vi "RSZVB Select Y-Parameters.vi"(4 "Out Mode (0: Single-ended (for unbalanced ports))":u16(ring) items=["Single-ended", "Differential", "Common"], 5 "In Port (1)":i32=1, 6 "In Mode (0: Single-ended (for unbalanced ports))":u16(ring) items=["Single-ended", "Differential", "Common"], 7 "Out Port (1)":i32=1, 8 "error in (no error)":errorcluster {"code" format="%.0x"}, 9 "Trace Name (Trc1)":string="Trc1", 10 "Channel (1)":i32=1, 11 "VISA session":refnum<visa-resource-name>) -> (0 "error out":errorcluster {"code" format="%.0x"}, 3 "dup VISA session":refnum<visa-resource-name>)   [LabVIEW 2011]
doc: "This VI select short-circuit Y-parameters for multiport measurements (including the 2-port Y-parameters) or mixed mode Y-parameters. All possible combinations of mixed mode parameters (e.g. Yss, Ycs, Yds, Ydd,...) are provided.\n\nAssigns a measurement parameter to an existing trace or creates a trace and assigns a channel number, a name and a measurement parameter to it. The trace is not displayed.\n\nMixed mode parameters are used to distinguish the following three port modes: \n\nSingle-ended (for unbalanced ports)\nDifferential mode (for balanced ports)\nCommon mode (for balanced ports) \n\nThe notation of a general Y-parameter is Y<mout><min><out><in>, where <mout> and <min> denote the output and input port modes, <out> and <in> denote the output and input port numbers.\n\nThe selected modes must be compatible with the port configuration. If an attempt is made to select an incompatible parameter (e.g. a single-ended parameter for a balanced port), the analyzer displays an error message.\n\nRemote-control command(s):\nCALCulate<Ch>:PARameter:SDEFine '<string>', 'Y11' | 'Y12' | 'Y21' | 'Y22' | ...\nCALCulate<Ch>:PARameter:MEASure '<string>', 'Y11' | 'Y12' | 'Y21' | 'Y22' | ..."
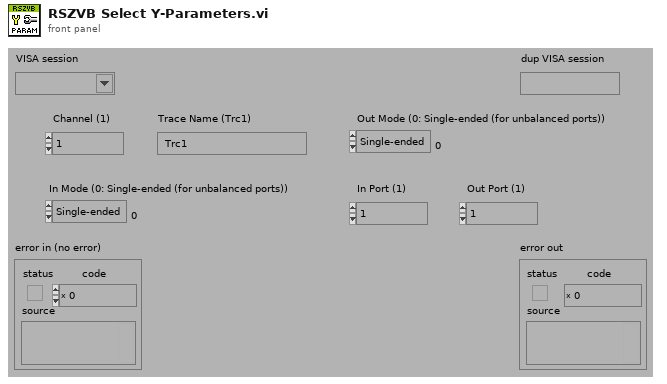
[diagram p1: front panel]
types:
  T1 = cluster{"Error Checking (T: On)":bool, "Installed Options":string[], "Data Valid?":bool, "Ports":i32, "Model":string[], "Option Checking (T: On)":bool}
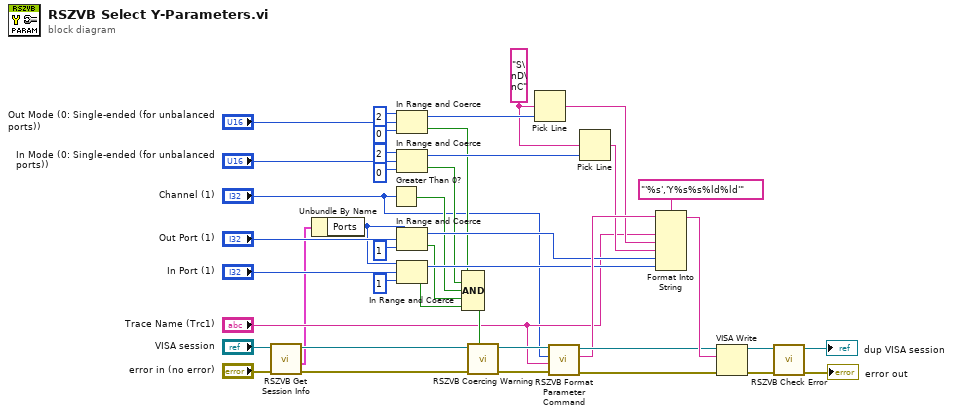
[diagram p0: block diagram]
diagram:
  w16 = "S\nD\nC"
  n1 = call "RSZVB Get Session Info.vi"("error in (no error)"="error in (no error)", "VISA session"="VISA session") -> ("error out"=w4:errorcluster, "Session Info"=w2:T1, "dup VISA session"=w3:refnum<visa-resource-name>)  [unwired: 7 in]
  n2 = Unbundle By Name(w2) -> ("Ports"=w1:i32)
  n3 = Greater Than 0?(x="Channel (1)") -> (x > 0?=w19:bool)
  n4 = In Range and Coerce(upper limit=u16 2, x="Out Mode (0: Single-ended (for unbalanced ports))", lower limit=u16 0) -> (coerced(x)=w27:u16, In Range?=w21:bool)
  n5 = In Range and Coerce(upper limit=u16 2, x="In Mode (0: Single-ended (for unbalanced ports))", lower limit=u16 0) -> (coerced(x)=w26:u16, In Range?=w20:bool)
  n6 = In Range and Coerce(upper limit=w1, x="Out Port (1)", lower limit=1) -> (coerced(x)=w23:i32, In Range?=w18:bool)
  n7 = In Range and Coerce(upper limit=w1, x="In Port (1)", lower limit=1) -> (coerced(x)=w22:i32, In Range?=w17:bool)
  n8 = Compound Arithmetic op=AND(w21, w20, w19, w18, w17) -> (w38:bool)
  n9 = call "RSZVB Coercing Warning.vi"("In Range?"=w38, "error in (no error)"=w4, "VISA session"=w3) -> ("error out"=w35:errorcluster, "dup VISA session"=w34:refnum<visa-resource-name>)  [unwired: 7 in]
  n10 = Pick Line(multi-line string=w16, line index=w27) -> (output string=w25:string)  [unwired: 1 in]
  n11 = call "RSZVB Format Parameter Command.vi"("error in (no error)"=w35, "Trace Name (Trc1)"="Trace Name (Trc1)", "Channel (1)"="Channel (1)", "VISA session"=w34) -> ("error out"=w36:errorcluster, "Buffer"=w30:string, "dup VISA session"=w33:refnum<visa-resource-name>)  [unwired: 5 in]
  n12 = Pick Line(multi-line string=w16, line index=w26) -> (output string=w24:string)  [unwired: 1 in]
  n13 = Format Into String(format string="'%s','Y%s%s%ld%ld'", initial string=w30, "Trace Name (Trc1)", w25, w24, w23, w22) -> (resulting string=w37:string)  [unwired: 1 in, 1 out]
  n14 = VISA Write(VISA resource name=w33, write buffer=w37, error in (no error)=w36) -> (VISA resource name out=w39:refnum<visa-resource-name>, error out=w40:errorcluster)  [unwired: 1 out]
  n15 = call "RSZVB Check Error.vi"("error in (no error)"=w40, "VISA session"=w39) -> ("error out"=→"error out":errorcluster, "dup VISA session"=→"dup VISA session":refnum<visa-resource-name>)  [unwired: 8 in]
